vi "softtrigger_final.vi"(8 "error in (no error)":errorcluster, 9 "TriggerRate":u8(ring)=4 items=["125Hz", "250Hz", "500Hz", "1000Hz", "2000Hz", "4000Hz", "5000Hz", "10000Hz", "20000Hz", "50000Hz"], 10 "SoftTrigger":bool=TRUE, 11 "address":string="192.168.10.35") -> (0 "error out":errorcluster)   [LabVIEW 2017]
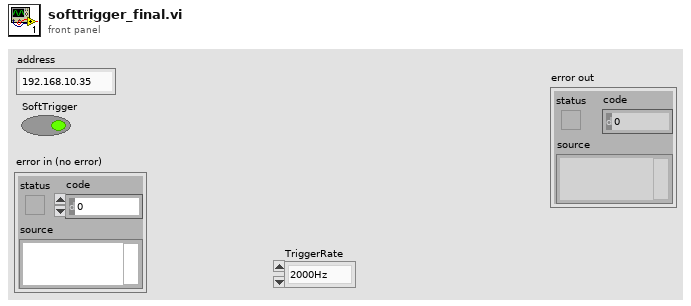
[diagram p1: front panel]
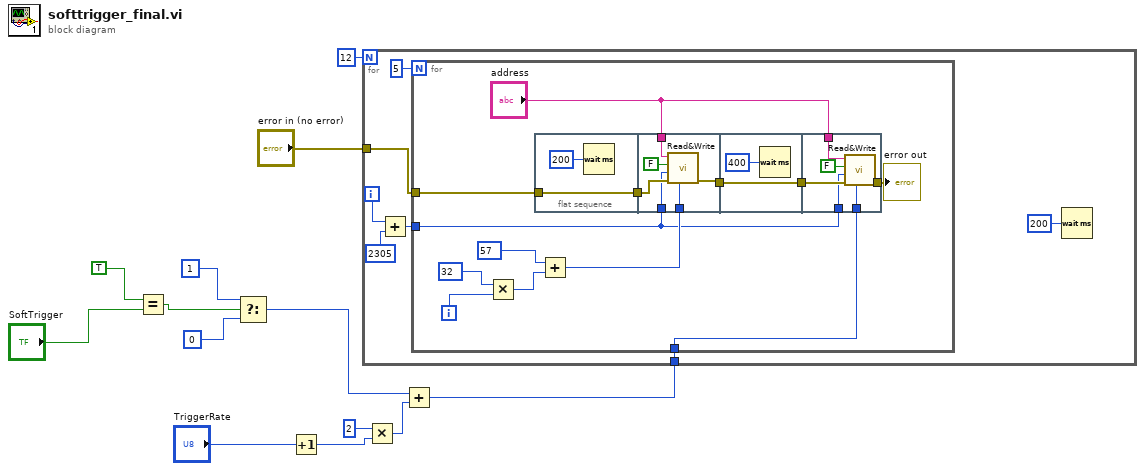
[diagram p0: block diagram]
diagram:
  n1 = Equal?(x=TRUE, y="SoftTrigger") -> (x = y?=w12:bool)
  n2 = Select(t=u8 1 ("In 3"), s=w12, f=u8 0 ("In 3")) -> (s? t:f=w6:u8)
  n3 = Increment(x="TriggerRate") -> (x+1=w3:u8)
  n4 = Multiply(x=u8 2, y=w3) -> (x*y=w5:u8)
  n5 = Add(x=w6, y=w5) -> (x+y=w7:u8)
  n6 = for {
    N: 12 -> [_]
    tunnel: w7 -> [w20]
    tunnel: "error in (no error)" -> [w16]
    i -> [w17]
    n7 = Add(x=w17, y=u32 2305 ("Address")) -> (x+y=w15:u32)
    n8 = for {
      N: 5 -> [_]
      tunnel: w20 -> [w32]
      tunnel: w16 -> [w24]
      tunnel: w15 -> [w23]
      i -> [w28]
      n9 = Multiply(x=u8 32 ("In"), y=w28) -> (x*y=w29:i32)
      n10 = flat-sequence {
        tunnel: w24 -> [w35]
        tunnel: [w35] -> w21
        tunnel: [w36] -> w26
        tunnel: w25 -> [w41]
        tunnel: w23 -> [w39]
        tunnel: "address" -> [w37]
        tunnel: w21 -> [w40]
        tunnel: [w43] -> w27
        tunnel: w26 -> [w43]
        tunnel: "address" -> [w47]
        tunnel: [w46] -> w33
        tunnel: w32 -> [w45]
        tunnel: w23 -> [w44]
        tunnel: w27 -> [w49]
        frame #0 {
          n11 = Wait (ms)(milliseconds to wait=u32 200 ("等待时间（毫秒）")) -> ()  [unwired: 1 out]
        }
        frame #1 {
          n12 = call "Read&Write.vi"("In"=w41, "error in (no error)"=w40, "Address"=w39, "Read (TRUE)"=FALSE, "address"=w37) -> ("error out"=w36:errorcluster)  [unwired: 5 in, 1 out]
        }
        frame #2 {
          n13 = Wait (ms)(milliseconds to wait=u32 400 ("等待时间（毫秒）")) -> ()  [unwired: 1 out]
        }
        frame #3 {
          n14 = call "Read&Write.vi"("In"=w45, "error in (no error)"=w49, "Address"=w44, "Read (TRUE)"=FALSE, "address"=w47) -> ("error out"=w46:errorcluster)  [unwired: 5 in, 1 out]
        }
      }
      n15 = Add(x=u8 57 ("In"), y=w29) -> (x+y=w25:i32)
      "error out" <- w33
    }
    n16 = Wait (ms)(milliseconds to wait=u32 200 ("等待时间（毫秒）")) -> ()  [unwired: 1 out]
  }
